vi "Helmholtz2D_FEM_Delaunay_Check Tri.vi"(7 "Angle":cluster{"angle":dbl, "y":i32}[](array[cluster]), 8 "Triangles In":i32[][](array[numeric]), 9 "Index":i32[](array[numeric]), 10 "Y":dbl[](array[numeric]), 11 "X":dbl[](array[numeric])) -> (0 "Triangles Out":i32[][](array[numeric]), 1 "new index":i32, 2 "Y Out":dbl[](array[numeric]), 3 "X Out":dbl[](array[numeric]))   [LabVIEW 2017, in "NI_PDE.lvlib"]
uses:
  <vilib>/gmath/NI_PDE.lvlib
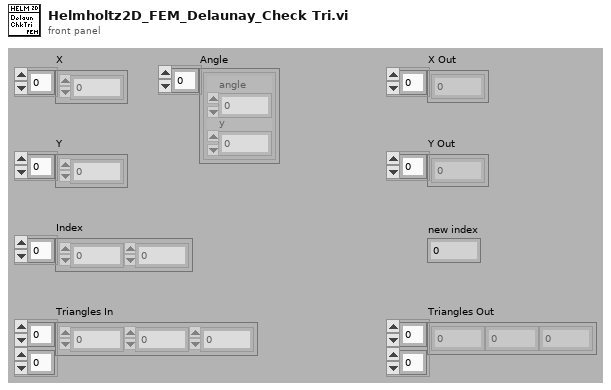
[diagram p1: front panel]
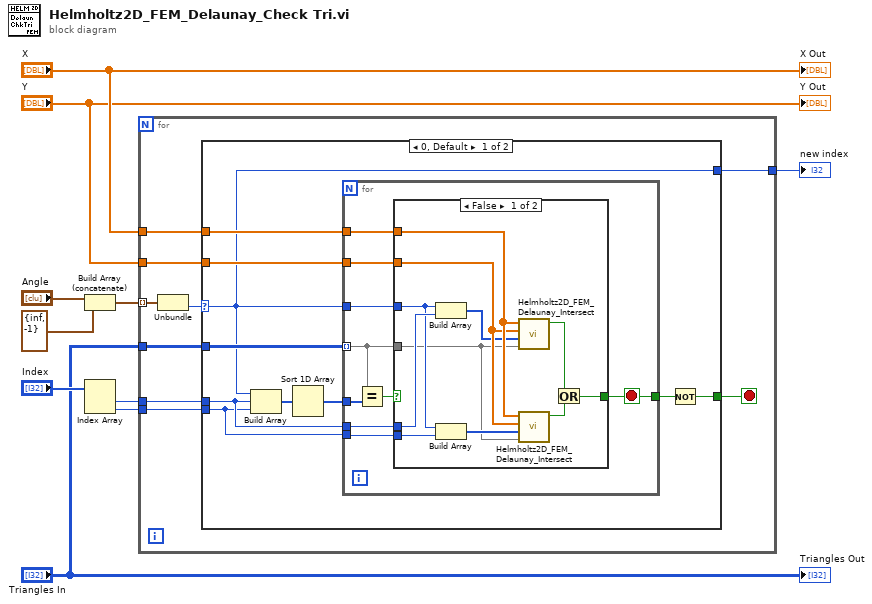
[diagram p0: block diagram]
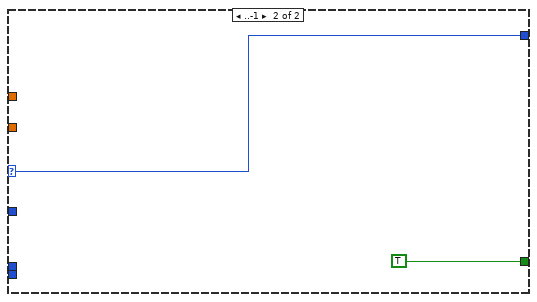
[diagram p3: hidden frame]
diagram:
  n1 = Build Array (concatenate)("Angle", cluster{"angle":dbl, "y":i32} {"angle"=inf, "y"=-1}) -> (w7:cluster{"angle":dbl, "y":i32}[])
  n2 = Index Array(array="Index") -> (element #1=w10:i32, element #2=w9:i32)  [unwired: 2 in]
  n3 = for {
    tunnel: w7 -> [w19] mode=indexing
    tunnel: "Triangles In" -> [w17]
    tunnel: w10 -> [w16]
    tunnel: w9 -> [w15]
    tunnel: "X" -> [w14]
    tunnel: "Y" -> [w13]
    tunnel: [w11] -> w2
    stop <- w12 stop-if-true
    n4 = Unbundle(w19) -> ("y"=w18:i32)  [unwired: 1 out]
    n5 = case shown="0, Default" w18 {
      selector: w18 -> [w20 w51]
      tunnel: w17 -> [w29 _]
      tunnel: w16 -> [w25 _]
      tunnel: w15 -> [w24 _]
      tunnel: w14 -> [w28 _]
      tunnel: w13 -> [w27 _]
      tunnel: [w21 TRUE] -> w12
      tunnel: [w20 w51] -> w11
      frame 0, Default {
        n6 = Build Array(w20, w25, w24) -> (w26:i32[])
        n7 = Sort 1D Array(array=w26) -> (sorted array=w23:i32[])
        n8 = for {
          tunnel: w29 -> [w34] mode=indexing
          tunnel: w20 -> [w37]
          tunnel: w25 -> [w36]
          tunnel: w24 -> [w35]
          tunnel: w28 -> [w33]
          tunnel: w27 -> [w32]
          tunnel: [w31] -> w22
          tunnel: w23 -> [w30]
          stop <- w31 stop-if-true
          n9 = Equal?(x=w34, y=w30) -> (x = y?=w38:bool)
          n10 = case shown="False" w38 {
            selector: w38 -> [_ w50]
            tunnel: w37 -> [w47 _]
            tunnel: w36 -> [w49 _]
            tunnel: w35 -> [w48 _]
            tunnel: w34 -> [w39 _]
            tunnel: w33 -> [w46 _]
            tunnel: w32 -> [w45 _]
            tunnel: [w42 w50] -> w31
            frame False {
              n11 = Build Array(w47, w49) -> (w41:i32[])
              n12 = Build Array(w47, w48) -> (w40:i32[])
              n13 = call <vilib>:"Helmholtz2D_FEM_Delaunay_Intersect.vi"("Triangle"=w39, "Index"=w41, "Y"=w45, "X"=w46) -> ("intersect?"=w44:bool)  [unwired: 7 out]
              n14 = call <vilib>:"Helmholtz2D_FEM_Delaunay_Intersect.vi"("Triangle"=w39, "Index"=w40, "Y"=w45, "X"=w46) -> ("intersect?"=w43:bool)  [unwired: 7 out]
              n15 = Or(x=w44, y=w43) -> (x .or. y?=w42:bool)
            }
            frame True {
              # "This triangle is already found."
            }
          }
        }
        n16 = Not(x=w22) -> (.not. x?=w21:bool)
      }
      frame ..-1 {
      }
    }
  }
  "new index" <- w2
  "X Out" <- "X"
  "Y Out" <- "Y"
  "Triangles Out" <- "Triangles In"
